vi "Send Response.vi"(6 "overwrite on timeout (T)":bool, 8 "error in (no error)":errorcluster, 9 "timeout in ms (0)":i32, 10 "response":T1, 11 "Interface in":refnum<class "Interface.lvclass">) -> (0 "error out":errorcluster, 1 "timed out?":bool, 3 "Interface out":refnum<class "Interface.lvclass">)   [LabVIEW 2017, in "DSF Core.lvlib" / "Interface.lvclass"]
uses:
  Interface.lvclass
  RT FIFO Data.ctl
  RT FIFO Parameters.ctl
  Interface.lvclass/Interface.ctl
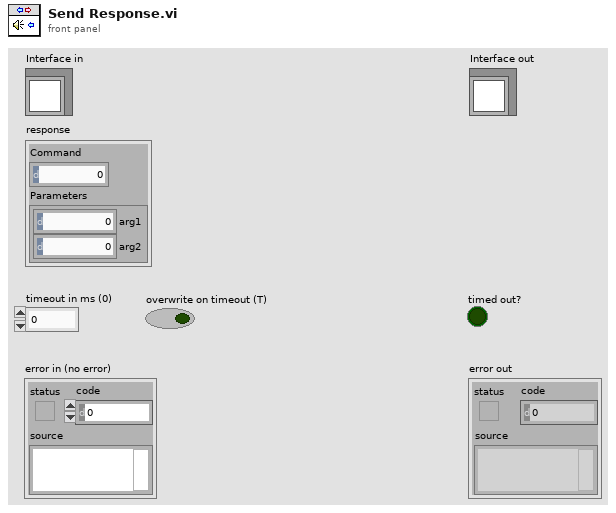
[diagram p1: front panel]
types:
  T1 = typedef "DSF Core.lvlib/Interface.lvclass/RT FIFO Data.ctl" = cluster{"Command":u8, "Parameters":T2}
  T2 = typedef "DSF Core.lvlib/Interface.lvclass/RT FIFO Parameters.ctl" = cluster{"arg1":u64, "arg2":u64}
  T3 = typedef "DSF Core.lvlib/DSF FIFO Options.ctl" = cluster{"Infinite Timeouts":bool}
  T4 = typedef "DSF Core.lvlib/Interface.lvclass/RT FIFO Ref.ctl" = refnum<k33>
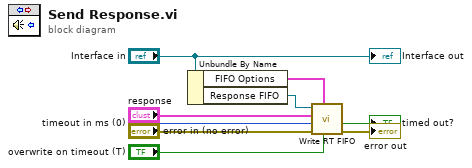
[diagram p0: block diagram]
diagram:
  n1 = Unbundle By Name("Interface in") -> ("FIFO Options"=w1:T3, "Response FIFO"=w2:T4)
  n2 = call "Write RT FIFO.vi"("overwrite on timeout (T)"="overwrite on timeout (T)", "FIFO Options"=w1, "error in (no error)"="error in (no error)", "timeout in ms (0)"="timeout in ms (0)", "element"="response", "RT FIFO in"=w2) -> ("error out"=→"error out":errorcluster, "timed out?"=→"timed out?":bool)  [unwired: 3 in, 1 out]
  "Interface out" <- "Interface in"
